vi "WAIT.vi"(9 "error in (no error)":errorcluster, 13 "Time to wait":dbl) -> (10 "error out":errorcluster)   [LabVIEW 2017]
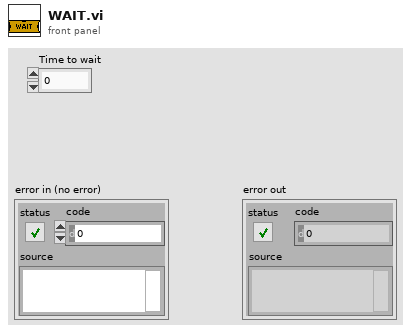
[diagram p1: front panel]
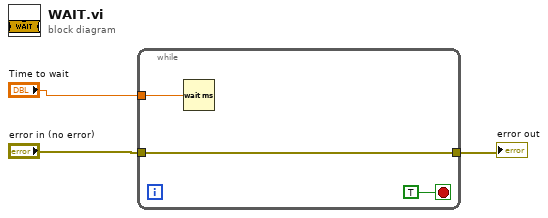
[diagram p0: block diagram]
diagram:
  n1 = while {
    tunnel: "Time to wait" -> [w5]
    tunnel: "error in (no error)" -> [w4]
    tunnel: [w4] -> w1
    stop <- TRUE stop-if-true
    n2 = Wait (ms)(milliseconds to wait=w5) -> ()  [unwired: 1 out]
  }
  "error out" <- w1
